vi "BroadcastIndividualStatusData.vi"(4 "error in":errorcluster, 5 "Robot Input & Status":T1={"Left PWM"=1500, "Right PWM"=1500, "Robot Heading"=0, "UDP Transmitting Port"=0, "UDP Receiving Port"=0, "Robot Symbol"=""}, 6 "Transmission Port":i32, 7 "Connection ID":refnum<k16>) -> (0 "error out":errorcluster, 1 "Right PWM":i32, 2 "Left PWM":i32, 3 "Connection ID":refnum<k16>)   [LabVIEW 2012]
panel:
  out "Robot Input":cluster{"Header":string, i32, i32}
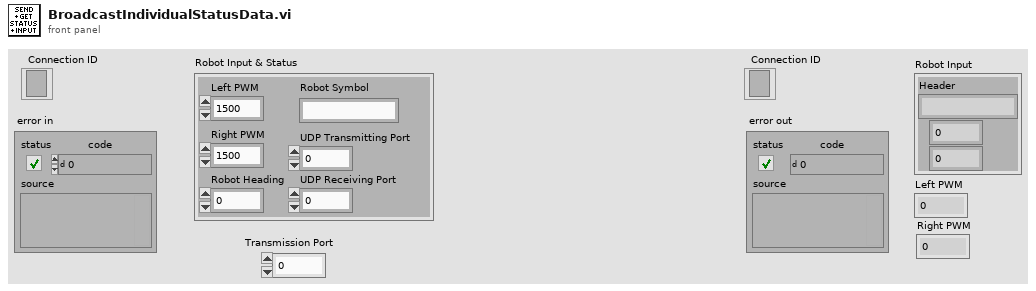
[diagram p1: front panel]
types:
  T1 = cluster{"Left PWM":i32, "Right PWM":i32, "Robot Heading":i32, "UDP Transmitting Port":i32, "UDP Receiving Port":i32, "Robot Symbol":string}
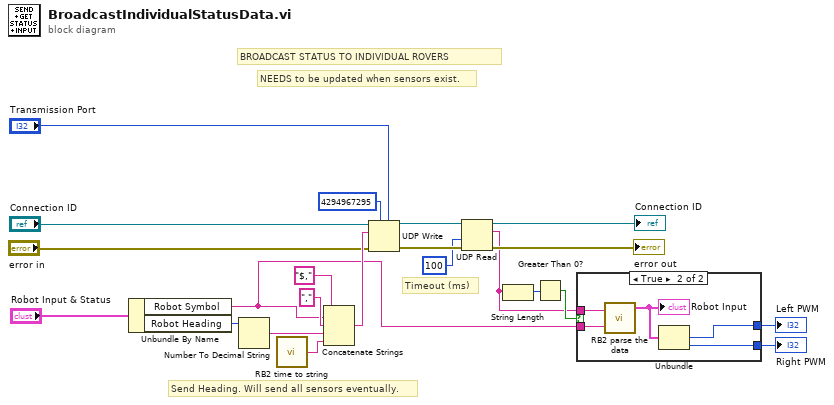
[diagram p0: block diagram]
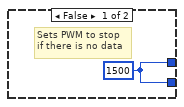
[diagram p2: hidden frame]
diagram:
  # "Timeout (ms)"
  # "Send Heading. Will send all sensors eventually."
  # "NEEDS to be updated when sensors exist."
  # "BROADCAST STATUS TO INDIVIDUAL ROVERS"
  n1 = Unbundle By Name("Robot Input & Status") -> ("Robot Symbol"=w12:string, "Robot Heading"=w21:i32)
  n2 = Number To Decimal String(number=w21) -> (decimal integer string=w19:string)  [unwired: 1 in]
  n3 = call "RB2 time to string.vi"() -> ("time string"=w20:string)  [unwired: 1 in]
  n4 = Concatenate Strings("$," ("string"), w12, "," ("string"), w19, w20) -> (w16:string)
  n5 = UDP Write(address=u32 4294967295, port or service name="Transmission Port", connection ID="Connection ID", data in=w16, 8:"error in") -> (error out=w14:errorcluster, 3:w15:refnum<k16>)  [unwired: 1 in]
  n6 = UDP Read(connection ID=w15, timeout ms (25000)=100, 8:w14) -> (data out=w1:string, error out=→"error out":errorcluster, 3:→"Connection ID":refnum<k16>)  [unwired: 1 in, 2 out]
  n7 = String Length(string=w1) -> (length=w2:i32)
  n8 = Greater Than 0?(x=w2) -> (x > 0?=w3:bool)
  n9 = case shown="True" w3 {
    tunnel: w12 -> [_ w28]
    tunnel: [w23 w26] -> w5
    tunnel: [w23 w25] -> w4
    tunnel: w1 -> [_ w24]
    frame False {
      w23 = 1500
      # "Sets PWM to stop\nif there is no data"
    }
    frame True {
      n10 = call "RB2 parse the data.vi"("Nav String"=w24, "Jeep"=w28) -> ("Jeep Data"=w27:cluster{"Header":string, i32, i32})  [unwired: 2 out]
      "Robot Input" <- w27
      n11 = Unbundle(w27) -> (w26:i32, w25:i32)  [unwired: 1 out]
    }
  }
  "Left PWM" <- w5
  "Right PWM" <- w4
